vi "Apply Wheel State.vi"(8 "error in (no error)":errorcluster, 10 "wheel state in":T1, 11 "caster wheel in":refnum<class "NI_Robotics_Caster Wheel.lvclass">) -> (0 "error out":errorcluster, 2 "wheel state out":T1, 3 "caster wheel out":refnum<class "NI_Robotics_Caster Wheel.lvclass">)   [LabVIEW 2017, in "NI_Robotics_Caster Wheel.lvclass"]
uses:
  <vilib>/robotics/Steering/Caster Wheel/NI_Robotics_Caster Wheel.lvclass
  c:/Program Files (x86)/National Instruments/LabVIEW 2017/vi.lib/robotics/Steering/Wheel/NI_Robotics_Wheel.lvclass
  <vilib>/robotics/Steering/Wheel/Wheel State.ctl
  <vilib>/robotics/Steering/Wheel/NI_Robotics_Wheel.lvclass/NI_Robotics_Wheel.ctl
  <vilib>/robotics/Steering/Caster Wheel/NI_Robotics_Caster Wheel.lvclass/NI_Robotics_Caster Wheel.ctl
  <vilib>/robotics/Actuation/Motor Communication/Update Motor Velocity Setpoint.vi
  <vilib>/robotics/Actuation/Motor Communication/Check if Valid.vi
  <vilib>/robotics/Utilities/Generate Error.vi
  <vilib>/robotics/Actuation/Motor Communication/NI_Robotics_Motor Communication.lvclass
  <vilib>/robotics/Steering/Wheel/NI_Robotics_Wheel.lvclass
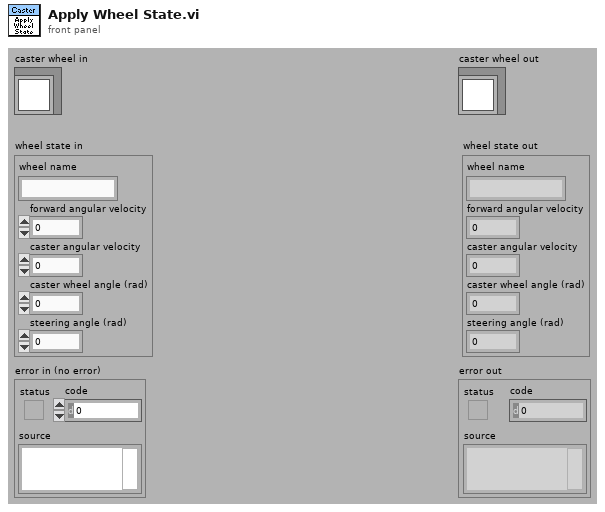
[diagram p1: front panel]
types:
  T1 = typedef "NI_Robotics_Wheel.lvclass/Wheel State.ctl" = cluster{"wheel name":string, "forward angular velocity":dbl, "caster angular velocity":dbl, "caster wheel angle (rad)":dbl, "steering angle (rad)":dbl}
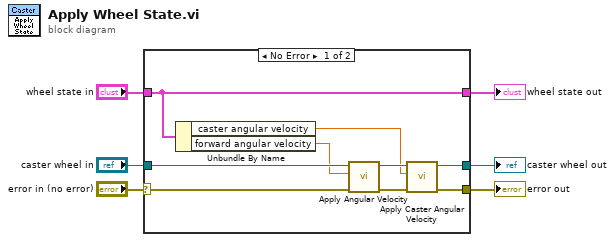
[diagram p0: block diagram]
diagram:
  n1 = case shown="No Error" "error in (no error)" {
    selector: "error in (no error)" -> [w15 w17]
    tunnel: "caster wheel in" -> [w14 w18]
    tunnel: "wheel state in" -> [w9 w16]
    tunnel: [w10 w18] -> w3
    tunnel: [w11 w17] -> w2
    tunnel: [w9 w16] -> w1
    frame No Error {
      n2 = Unbundle By Name(w9) -> ("caster angular velocity"=w8:dbl, "forward angular velocity"=w7:dbl)
      n3 = call <vilib>:"Apply Angular Velocity.vi"("error in (no error)"=w15, "forward angular velocity"=w7, "wheel in"=w14) -> ("error out"=w13:errorcluster, "wheel out"=w12:refnum<class "NI_Robotics_Caster Wheel.lvclass">)  [unwired: 7 in]
      n4 = call <vilib>:"Apply Caster Angular Velocity.vi"("error in (no error)"=w13, "caster angular velocity"=w8, "caster wheel in"=w12) -> ("error out"=w11:errorcluster, "caster wheel out"=w10:refnum<class "NI_Robotics_Caster Wheel.lvclass">)  [unwired: 7 in]
    }
    frame Error {
    }
  }
  "error out" <- w2
  "caster wheel out" <- w3
  "wheel state out" <- w1
